vi "CV_main.vi"(0 "Start bias":dbl=-8.0, 1 "End bias":dbl=1.0, 2 "Bias step":dbl=0.25, 3 "Delay time":dbl=250.0, 4 "# scans":dbl=50.0, 5 "Error In":errorcluster, 6 "Hardware GPIB address":string="18") -> (14 "CV":cluster{dbl[], dbl[]}(graph), 15 "1/C2":cluster{dbl[], dbl[]}(graph), 16 "GV":cluster{dbl[], dbl[]}(graph), 17 "Target vs Real Bias":cluster{dbl[], dbl[]}(graph), 19 "Error Out":errorcluster)   [LabVIEW 2015, in "CV.lvlib"]
uses:
  CV.lvlib
  Hardware libraries/Boonton7200/Boonton7200_Special_Function_Codes.ctl
  Hardware libraries/Boonton7200/Boonton7200_IEEE-488_Bus_Mnemonics.ctl
  Hardware libraries/Boonton7200/Boonton7200.lvlib
panel:
  out "Live Plot":cluster{"X":dbl, "Y":dbl}[](graph)
  in  "Capacitance Range":T1=enum."Set and hold 20.00 pF / 20.0 uS range"
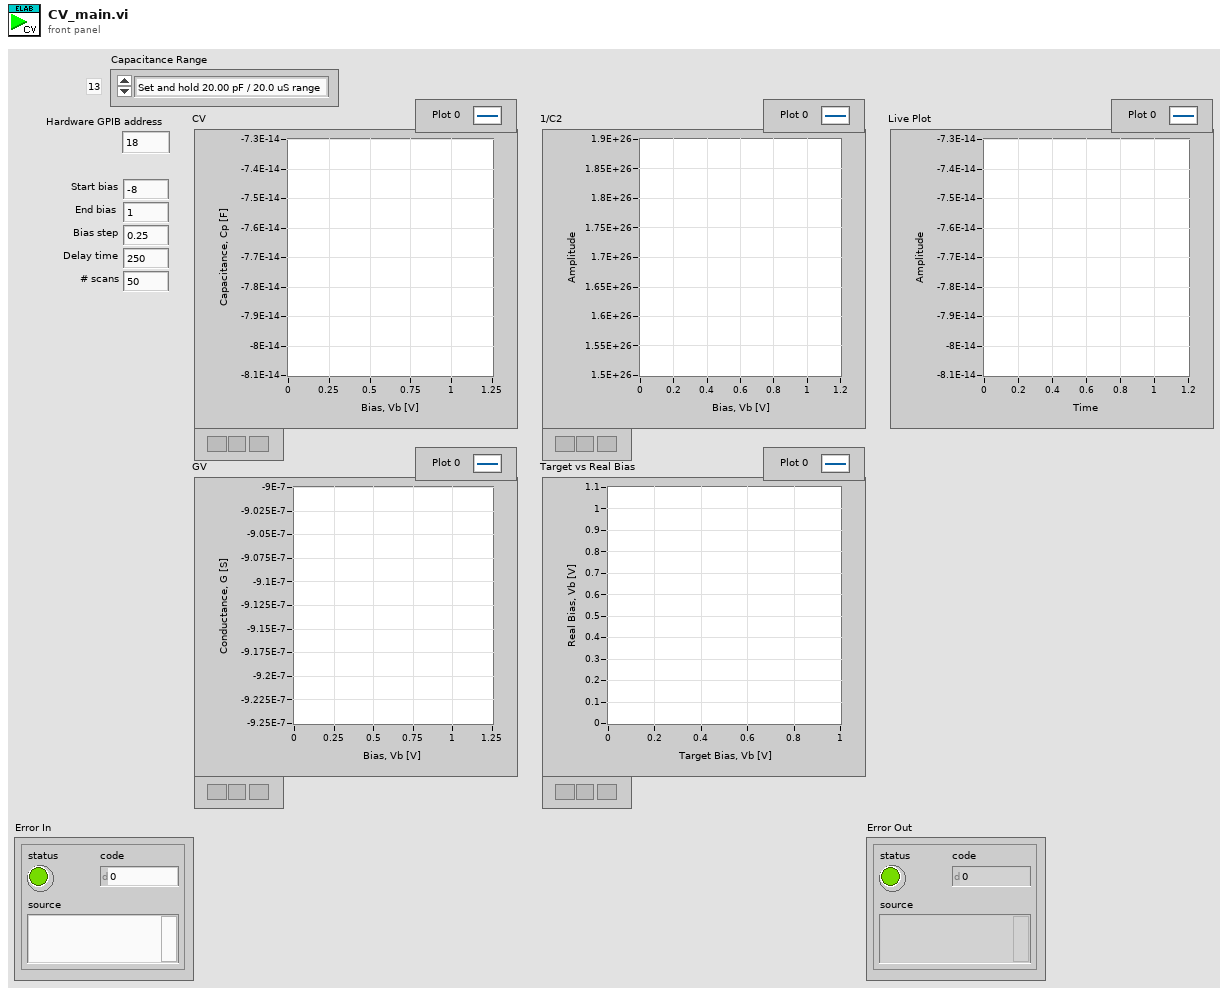
[diagram p1: front panel]
types:
  T1 = typedef "Boonton7200_Special_Function_Codes.ctl" = enum16{"Execute special functions 10,20,30 and 40", "Test Level display and entry", "Capacitance Standard display and entry", "Conductance Standard dispaly and entry", "Capacitance Low Limit display and entry", "Capacitance High Limit dispaly and entry", "IEEE-488 Bus Address display and entry", "End-of-string charecter display and selection", "Capacitance uncertainty display", "Conductance uncertainty dispaly", "Automatic selection(Measurement Ranging Functions)", "Hold current measurement range", "Set and hold 2.000 pF / 2.00 uS range", "Set and hold 20.00 pF / 20.0 uS range", "Set and hold 200.0 pF / 200 uS range", "Set and holde 2000 pF / 2000 uS range", "16 - Not Defined", "17 - Not Defined", "18 - Not Defined", "19 - Not Defined", "Automatic selection(Internal Bias Ranging Functions)", "Hold current bias range", "Set and hold 20.000 V range", "Set and Hold 100.00 V range", "24 - Not Defined", "25 - Not Defined", "26 - Not Defined", "27 - Not Defined", "28 - Not Defined", "29 - Not Defined", "30 Automatic selection(Measurement Filter Functions)", "Filter length = 1 measurement, no average", "Filter length = 2 measurement", "Filter length = 5 measurement", "Filter length = 10 measurement", "Filter length = 20 measurement", "Filter length = 50 measurement", "Filter length = 100 measurement", "Filter length = 200 measurement", "Filter length = 500 measurement", "Normal operation, free-run dispaly(Sercvice Request Functions)", "Disable SRQ interrupt", "Enable SRQ interrupt", "Set SRQ mask when an error occurs", "Set SRQ mask and update dispaly when measurement filter is complete", "Set SRQ mask when capacitance measurement is within the high and low limit settings", "Set SRQ mask when capacitance measurement exceeds the high or low limit settings", "Set SRQ mask when zero or calibration is complete", "Set SRQ mask when sweep is complete", "49 - Not Defined", "Calibrate detector offset(Automatic Calibration and Test Functions)", "Calibrate external bias offset", "Calibrate internal bias offset", "Calibrate full-scale capacitance", "Calibrate conductance phase", "Display internal temperature", "Display amplitude error due to temperature influence", "Display phase error due to temperature influence", "Initialize instrument and erase all program locations", "Initalize software calibration variables"}
  T2 = typedef "Boonton7200_IEEE-488_Bus_Mnemonics.ctl" = string
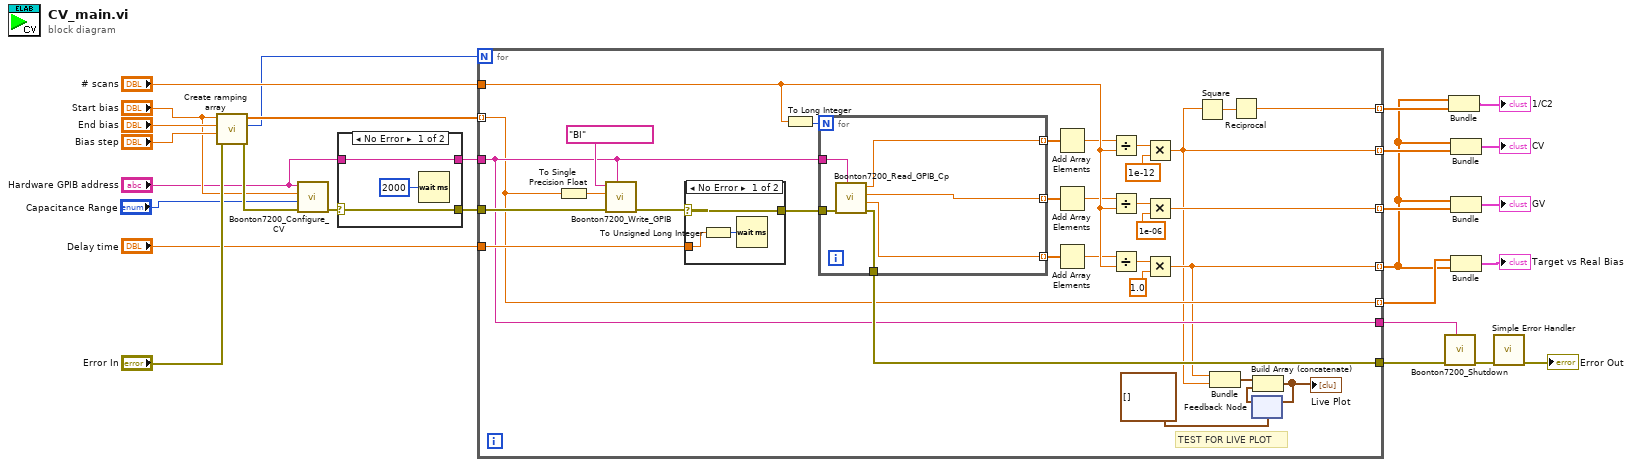
[diagram p0: block diagram]
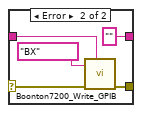
[diagram p2: hidden frame]
diagram:
  n1 = call "Create ramping array.vi"("Error In"="Error In", "Delta"="Bias step", "End"="End bias", "Start"="Start bias") -> ("Error Out"=w8:errorcluster, "Array length"=w16:i32, "Output Array (1D)"=w24:dbl[])  [unwired: 5 in]
  n2 = call "Boonton7200_Configure_CV.vi"("Error In"=w8, "Capacitance Range"="Capacitance Range", "Start Bias"="Start bias", "GPIB Address Sting"="Hardware GPIB address") -> ("Error Out"=w9:errorcluster)  [unwired: 7 in]
  n3 = case shown="No Error" w9 {
    selector: w9 -> [w30 w34]
    tunnel: [w30 w33] -> w18
    tunnel: [w28 "" ("Hardware GPIB address")] -> w12
    tunnel: "Hardware GPIB address" -> [w28 w32]
    frame No Error {
      n4 = Wait (ms)(milliseconds to wait=u32 2000) -> ()  [unwired: 1 out]
    }
    frame Error {
      n5 = call "Boonton7200_Write_GPIB.vi"("GPIB Address String"=w32, "Error In"=w34, "IEEE-488 Bus Mnemonics"=T2 "BX") -> ("Error Out"=w33:errorcluster)  [unwired: 8 in]
    }
  }
  n6 = for {
    N: w16 -> [_]
    tunnel: w18 -> [w52]
    tunnel: w24 -> [w44] mode=indexing
    tunnel: w12 -> [w45]
    tunnel: "Delay time" -> [w66]
    tunnel: "# scans" -> [w67]
    tunnel: [w41] -> w4 mode=indexing
    tunnel: [w42] -> w19 mode=indexing
    tunnel: [w40] -> w14 mode=indexing
    tunnel: [w53] -> w11
    tunnel: [w44] -> w5 mode=indexing
    tunnel: [w43] -> w13 mode=indexing
    tunnel: [w45] -> w10
    # "TEST FOR LIVE PLOT"
    n7 = To Single Precision Float(number=w44) -> (single precision float=w49:sgl)
    n8 = call "Boonton7200_Write_GPIB.vi"("GPIB Address String"=w45, "Error In"=w52, "Data Value"=w49, "IEEE-488 Bus Mnemonics"=T2 "BI") -> ("Error Out"=w50:errorcluster)  [unwired: 7 in]
    n9 = case shown="No Error" w50 {
      selector: w50 -> [w74 w77]
      tunnel: w66 -> [w75 _]
      tunnel: [w74 w77] -> w64
      frame No Error {
        n10 = To Unsigned Long Integer(number=w75) -> (unsigned 32bit integer=w76:u32)
        n11 = Wait (ms)(milliseconds to wait=w76) -> ()  [unwired: 1 out]
      }
      frame Error {
      }
    }
    n12 = To Long Integer(number=w67) -> (32bit integer=w65:i32)
    n13 = for {
      N: w65 -> [_]
      tunnel: w64 -> [w73]
      tunnel: w45 -> [w72]
      tunnel: [w68] -> w63 mode=indexing
      tunnel: [w69] -> w62 mode=indexing
      tunnel: [w70] -> w61 mode=indexing
      tunnel: [w71] -> w53
      n14 = call "Boonton7200_Read_GPIB_Cp.vi"("GPIB Address String"=w72, "Error In"=w73) -> ("Error Out"=w71:errorcluster, "External bias"=w70:dbl, "Conductance"=w69:dbl, "Capacitance"=w68:dbl)  [unwired: 5 in, 1 out]
    }
    n15 = Add Array Elements(numeric array=w63) -> (sum=w60:dbl)
    n16 = Add Array Elements(numeric array=w62) -> (sum=w59:dbl)
    n17 = Add Array Elements(numeric array=w61) -> (sum=w58:dbl)
    n18 = Divide(x=w60, y=w67) -> (x/y=w47:dbl)
    n19 = Divide(x=w59, y=w67) -> (x/y=w48:dbl)
    n20 = Divide(x=w58, y=w67) -> (x/y=w56:dbl)
    n21 = Multiply(x=w47, y=1e-12) -> (x*y=w40:dbl)
    n22 = Multiply(x=w48, y=1e-06) -> (x*y=w42:dbl)
    n23 = Multiply(x=w56, y=1.0) -> (x*y=w41:dbl)
    n24 = Square(x=w40) -> (x^2=w46:dbl)
    n25 = Bundle(w41, w40) -> (w38:cluster{dbl, dbl})  [unwired: 1 in]
    n26 = Reciprocal(x=w46) -> (1/x=w43:dbl)
    n27 = feedback #1(cluster{dbl, dbl}[] []) -> (w37:cluster{dbl, dbl}[])
    n28 = Build Array (concatenate)(w38, w37) -> (w39:cluster{dbl, dbl}[])
    "Live Plot" <- w39
    n29 = feedback-in #1(w39) -> ()
  }
  n30 = call "Boonton7200_Shutdown.vi"("GPIB Address String"=w10, "Error In"=w11) -> ("Error Out"=w2:errorcluster)  [unwired: 9 in]
  n31 = Bundle(w4, w13) -> (→"1/C2":cluster{dbl[], dbl[]})  [unwired: 1 in]
  n32 = Bundle(w4, w14) -> (→"CV":cluster{dbl[], dbl[]})  [unwired: 1 in]
  n33 = Bundle(w4, w19) -> (→"GV":cluster{dbl[], dbl[]})  [unwired: 1 in]
  n34 = Bundle(w5, w4) -> (→"Target vs Real Bias":cluster{dbl[], dbl[]})  [unwired: 1 in]
  n35 = call <vilib>:"Simple Error Handler.vi"("error in (no error)"=w2) -> ("error out"=→"Error Out":errorcluster)  [unwired: 4 in, 4 out]
